vi "Flatten.vi"(8 "error in (no error)":errorcluster, 11 "Msg in":refnum<class "Msg.lvclass">) -> (0 "error out":errorcluster, 2 "Buffer":u8[](array[numeric]) format="%.0x", 3 "Msg out":refnum<class "Msg.lvclass">)   [LabVIEW 2020, in "Discovery.lvlib" / "Msg.lvclass"]
uses:
  Msg.lvclass
  Msg.lvclass/Msg.ctl
  Discovery.lvlib
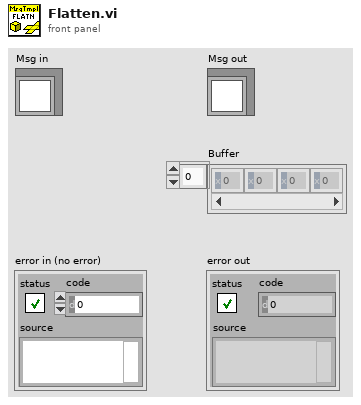
[diagram p1: front panel]
types:
  T1 = typedef "Discovery.lvlib/Data.ctl" = cluster{"Scalar":dbl, "Array":dbl[]}
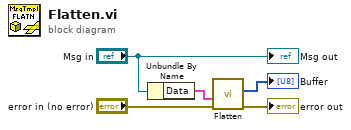
[diagram p0: block diagram]
diagram:
  n1 = Unbundle By Name("Msg in") -> ("Data"=w1:T1)
  n2 = call "Flatten.vi"("error in"="error in (no error)", "Data"=w1) -> ("error out"=→"error out":errorcluster, "Buffer"=→"Buffer":u8[])  [unwired: 8 in]
  "Msg out" <- "Msg in"
